vi "Teardown Init.vi"(7 "Is Sync":bool) -> (2 "Msg":refnum<class "Msg.lvclass">)   [LabVIEW 2021, in "jettl.lvlib" / "Teardown Msg.lvlib"]
uses:
  Teardown Msg.lvlib
  Msg/Msg.lvclass
  Teardown Msg/Teardown Msg.lvclass
  C:/git/jettl/jettl/jettl/Msg/Msg.lvclass
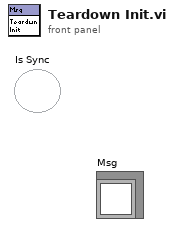
[diagram p1: front panel]
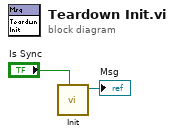
[diagram p0: block diagram]
diagram:
  n1 = call "Init.vi"("Is Sync"="Is Sync") -> ("Teardown Msg out"=→"Msg":refnum<class "Teardown Msg.lvclass">)  [unwired: 10 in]
